vi "Generate Docs.vi"(8 "error in (no error)":errorcluster, 10 "Files Generated by Build":path[](array[path]), 11 "Destination Path":path) -> (0 "error out":errorcluster)   [LabVIEW 2015]
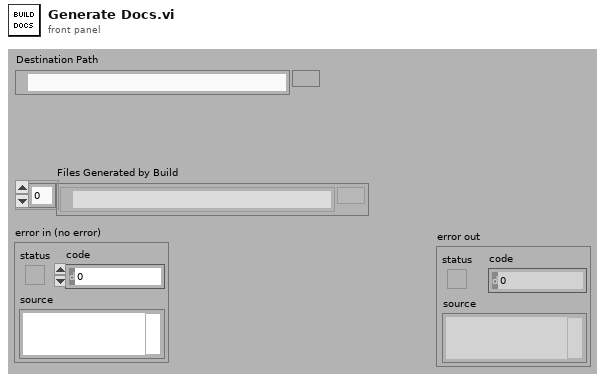
[diagram p1: front panel]
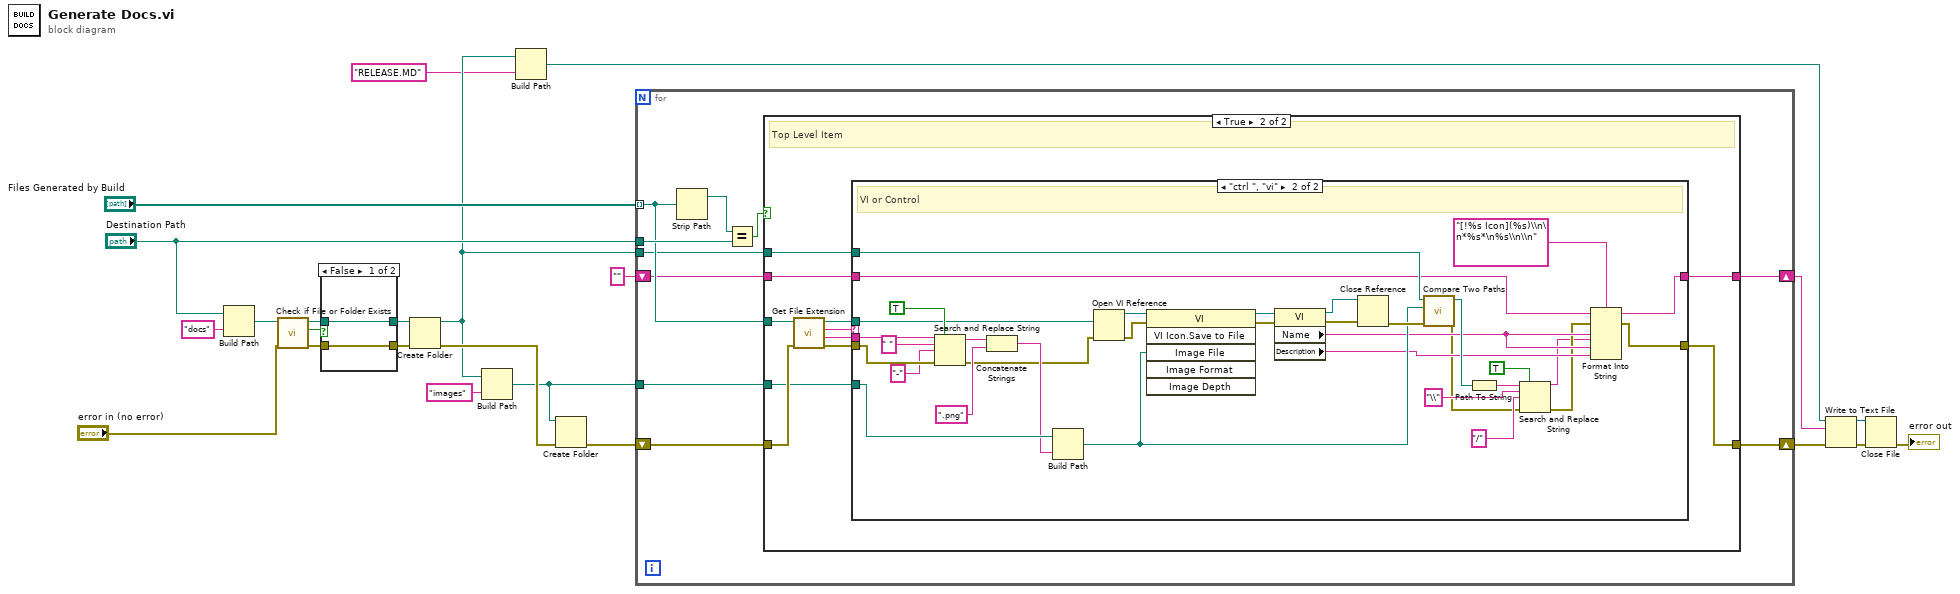
[diagram p0: block diagram]
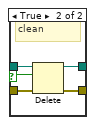
[diagram p2: hidden frame]
diagram:
  n1 = Build Path(base path="Destination Path", name or relative path="docs") -> (appended path=w22:path)
  n2 = call <vilib>:"Check if File or Folder Exists.vi"("error in (no error)"="error in (no error)", "path"=w22) -> ("error out"=w3:errorcluster, "file or folder exists?"=w1:bool, "dup path"=w4:path)  [unwired: 7 in]
  n3 = case shown="False" w1 {
    selector: w1 -> [_ w26]
    tunnel: [w25 w30] -> w21
    tunnel: [w24 w29] -> w20
    tunnel: w4 -> [w25 w28]
    tunnel: w3 -> [w24 w27]
    frame False {
    }
    frame True {
      # "clean"
      n4 = Delete(path (use dialog)=w28, entire hierarchy (F)=w26, error in=w27) -> (deleted path=w30:path, error out=w29:errorcluster)  [unwired: 2 in, 1 out]
    }
  }
  n5 = Create Folder(path (use dialog)=w21, error in=w20) -> (created path=w12:path, error out=w18:errorcluster)  [unwired: 1 in, 1 out]
  n6 = Build Path(base path=w12, name or relative path="images") -> (appended path=w16:path)
  n7 = Build Path(base path=w12, name or relative path="RELEASE.MD") -> (appended path=w6:path)
  n8 = Create Folder(path (use dialog)=w16, error in=w18) -> (error out=w17:errorcluster)  [unwired: 1 in, 2 out]
  n9 = for {
    shift-right: [w32] -> w10
    shift-left: w17 -> [w37]
    tunnel: w16 -> [w35]
    tunnel: "Destination Path" -> [w39]
    tunnel: "Files Generated by Build" -> [w36] mode=indexing
    shift-right: [w33] -> w5
    shift-left: "" -> [w34]
    tunnel: w12 -> [w31]
    n10 = Strip Path(path=w36) -> (stripped path=w40:path)  [unwired: 1 out]
    n11 = Equal?(x=w40, y=w39) -> (x = y?=w38:bool)
    n12 = case shown="True" w38 {
      tunnel: w37 -> [w41 w52]
      tunnel: w36 -> [_ w53]
      tunnel: w35 -> [_ w47]
      tunnel: w34 -> [w42 w46]
      tunnel: [w42 w45] -> w33
      tunnel: [w41 w44] -> w32
      tunnel: w31 -> [_ w43]
      frame False {
      }
      frame True {
        # "Top Level Item"
        n13 = call <vilib>:"Get File Extension.vi"("error in (no error)"=w52, "file"=w53) -> ("error out"=w49:errorcluster, "filename without extension"=w48:string, "lowercase file extension"=w51:string, "dup file"=w50:path)  [unwired: 5 in, 1 out]
        n14 = case shown="\"ctrl \", \"vi\"" w51 {
          tunnel: w50 -> [_ w80]
          tunnel: w49 -> [w54 w88]
          tunnel: w48 -> [_ w89]
          tunnel: w47 -> [_ w84]
          tunnel: w46 -> [w55 w66]
          tunnel: [w55 w65] -> w45
          tunnel: [w54 w64] -> w44
          tunnel: w43 -> [_ w71]
          frame Default {
            # "Skip"
          }
          frame "ctrl ", "vi" {
            # "VI or Control"
            n15 = Search and Replace String(replace all?=TRUE ("replace all? (F)"), input string=w89, search string=" ", replace string="-" ("replace string (\"\")"), error in=w88) -> (result string=w83:string, error out=w79:errorcluster)  [unwired: 3 in, 2 out]
            n16 = Concatenate Strings(w83, ".png" ("string")) -> (w81:string)
            n17 = Build Path(base path=w84, name or relative path=w81) -> (appended path=w70:path)
            n18 = Open VI Reference(vi path=w80, error in (no error)=w79) -> (vi reference=w78:refnum<vi>, error out=w77:errorcluster)  [unwired: 4 in]
            n19 = invoke class="VI" method="VI Icon.Save to File"(reference=w78, error in=w77, "Image File"=w70) -> (reference out=w76:refnum<vi>, error out=w75:errorcluster)  [unwired: 3 in, 4 out]
            n20 = property class="VI"(reference=w76, error in=w75) -> (reference out=w73:refnum<vi>, error out=w74:errorcluster, "Name"=w68:string, "Description"=w67:string)
            n21 = Close Reference(reference=w73, error in (no error)=w74) -> (error out=w72:errorcluster)
            n22 = call <vilib>:"Compare Two Paths.vi"("error in (no error)"=w72, "Path 2"=w70, "Path 1"=w71) -> ("error out"=w59:errorcluster, "Relative Path from 1 to 2"=w69:path)  [unwired: 5 in, 2 out]
            n23 = Path To String(path=w69) -> (string=w62:string)
            n24 = Search and Replace String(replace all?=TRUE ("replace all? (F)"), input string=w62, search string="\\", replace string="/" ("replace string (\"\")"), error in=w59) -> (result string=w56:string, error out=w58:errorcluster)  [unwired: 3 in, 2 out]
            n25 = Format Into String(format string="[!%s Icon](%s)\\n\n*%s*\n%s\\n\\n", initial string=w66, error in=w58, w68, w56, w68, w67) -> (resulting string=w65:string, error out=w64:errorcluster)
          }
        }
      }
    }
  }
  n26 = Write to Text File(file (use dialog)=w6, text=w5, error in=w10) -> (refnum out=w8:refnum<file>, error out=w9:errorcluster)  [unwired: 1 in, 1 out]
  n27 = Close File(refnum=w8, error in=w9) -> (error out=→"error out":errorcluster)  [unwired: 1 out]
